vi "TWM Client Open.vi"(7 "end of packet key":string="TWM:command:EndOfPacket", 8 "error in":errorcluster, 11 "pipe name":string="\\\\.\\pipe\\TWM:server" caption="Named Pipe Identifier") -> (0 "error out":errorcluster, 3 "handle out":i32)   [LabVIEW 2020, in "TWM Client.lvlib"]
doc: "Initialize TWM client. This will try to open named pipe to the TWM server. Note the server must exist first! Returns handle to the pipe which must not be lost. Do not forget to call TWM Client Close before exiting!"
uses:
  TWM Client.lvlib
  <vilib>/Utility/error.llb/Error Cluster From Error Code.vi
  <vilib>/ErrorRing/Error Ring.xnode
panel:
  out "TWM client version string":string
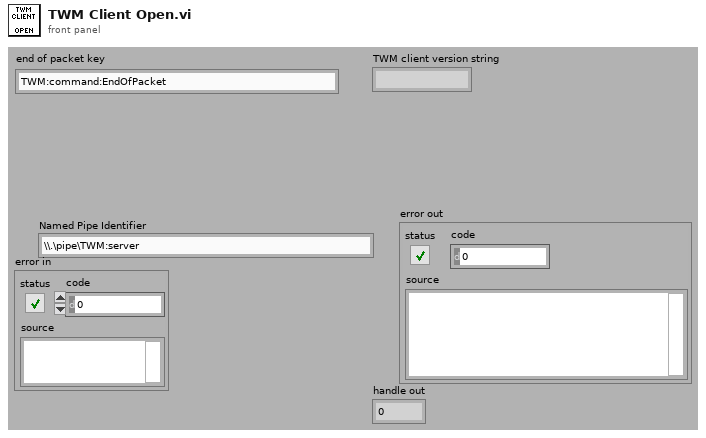
[diagram p1: front panel]
types:
  T1 = enum16{"CREATE_NEW", "CREATE_ALWAYS", "OPEN_EXISTING", "OPEN_ALWAYS", "TRUNCATE_EXISTING"}
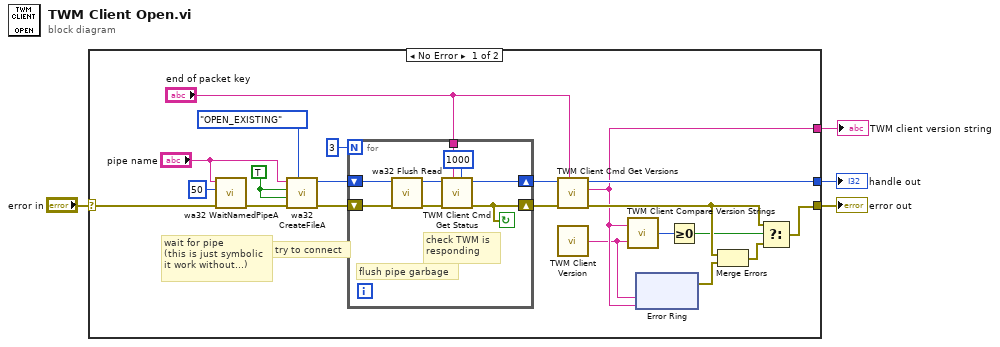
[diagram p0: block diagram]
diagram:
  n1 = case shown="No Error" "error in" {
    selector: "error in" -> [w18 w42]
    tunnel: [w10 w42] -> w4
    tunnel: [w15 _] -> w2
    tunnel: [w8 _] -> w1
    frame No Error {
      w25 = TRUE ("read")
      # "wait for pipe\n(this is just symbolic\nit work without...)"
      # "try to connect"
      n2 = call "wa32 WaitNamedPipeA.vi"("error in"=w18, "timeout [ms]"=u32 50, "pipe name"="pipe name") -> ("error out"=w23:errorcluster)  [unwired: 8 in]
      n3 = call "wa32 CreateFileA.vi"("creation dispozition"=T1."OPEN_EXISTING", "error in"=w23, "write"=w25, "read"=w25, "file path"="pipe name") -> ("error out"=w20:errorcluster, "handle"=w19:i32)  [unwired: 5 in]
      n4 = for {
        N: 3 -> [_]
        tunnel: "end of packet key" -> [w36]
        shift-right: [w35] -> w16
        shift-left: w20 -> [w41]
        shift-right: [w37] -> w14
        shift-left: w19 -> [w40]
        stop <- w35 continue-if-true
        # "check TWM is\nresponding"
        # "flush pipe garbage"
        n5 = call "wa32 Flush Read.vi"("error in"=w41, "handle"=w40) -> ("error out"=w39:errorcluster, "handle out"=w38:i32)  [unwired: 7 in, 1 out]
        n6 = call "TWM Client Cmd Get Status.vi"("timeout [ms] (3000)"=1000, "end of packet key"=w36, "error in"=w39, "handle"=w38) -> ("error out"=w35:errorcluster, "handle out"=w37:i32)  [unwired: 3 in, 3 out]
      }
      n7 = call "TWM Client Cmd Get Versions.vi"("end of packet key"="end of packet key", "error in"=w16, "handle"=w14) -> ("error out"=w11:errorcluster, "TWM client version string"=w8:string, "handle out"=w15:i32)  [unwired: 6 in]
      n8 = call "TWM Client Version.vi"() -> ("version string"=w7:string)
      n9 = call "TWM Client Compare Version Strings.vi"("version b"=w7, "version a"=w8) -> ("a>b, a=b, a<b {+1,0,-1}"=w6:i32)
      n10 = xnode ("Error Ring")("parameter 0"=w7, "parameter 1"=w8) -> ("error out"=w9:errorcluster)
      n11 = Greater Or Equal To 0?(x=w6) -> (x >= 0?=w5:bool)
      n12 = Merge Errors(w11, w9) -> (w12:errorcluster)
      n13 = Select(t=w11, s=w5, f=w12) -> (s? t:f=w10:errorcluster)
    }
    frame Error {
    }
  }
  "error out" <- w4
  "handle out" <- w2
  "TWM client version string" <- w1
